vi "myRIO_BRig_RT_dataTrial_laserPower_l2.vi"() -> (2 "output_laserPower_l2":i32)   [LabVIEW 2014]
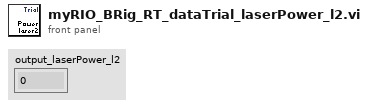
[diagram p1: front panel]
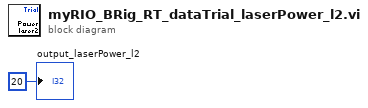
[diagram p0: block diagram]
diagram:
  "output_laserPower_l2" <- 20 ("output_iBlock")
